vi "Lab Panel V5.27.vi"() -> ()   [LabVIEW 2013] (continued)
                    n2201 = Unbundle By Name(w3868) -> ("OFF amps"=w3864:dbl, "VOLTS"=w3863:dbl, "PF"=w3862:dbl, "OFF amps"=w3861:dbl, "VOLTS"=w3860:dbl, "PF"=w3859:dbl)
                    n2202 = Unbundle By Name(w3865) -> ("1  (A) cal"=w3858:dbl, "1 (V) cal"=w3857:dbl, "1 (PF) cal"=w3856:dbl, "2 (A) cal"=w3855:dbl, "2 (V) cal"=w3854:dbl, "2 (PF) cal"=w3853:dbl)  [unwired: 4 out]
                    n2203 = Multiply(x=w3864, y=w3858) -> (x*y=w3851:dbl)
                    n2204 = Multiply(x=w3863, y=w3857) -> (x*y=w3850:dbl)
                    n2205 = Multiply(x=w3862, y=w3856) -> (x*y=w3849:dbl)
                    n2206 = Multiply(x=w3861, y=w3855) -> (x*y=w3847:dbl)
                    n2207 = Multiply(x=w3860, y=w3854) -> (x*y=w3846:dbl)
                    n2208 = Multiply(x=w3859, y=w3853) -> (x*y=w3845:dbl)
                    n2209 = local read "SIG LAB01-1"() -> (w3852:T2)
                    n2210 = local read "SIG LAB01-2"() -> (w3848:T2)
                    n2211 = Bundle By Name(cluster=w3852, "AMPS"=w3851, "VOLTS"=w3850, "PF"=w3849) -> (w3844:T2)
                    n2212 = Bundle By Name(cluster=w3848, "AMPS"=w3847, "VOLTS"=w3846, "PF"=w3845) -> (w3843:T2)
                    n2213 = global write "Global display 1.vi" "SIG LAB01-2"(w3843) -> ()
                    n2214 = global write "Global display 1.vi" "SIG LAB01-1"(w3844) -> ()
                    n2215 = local write "SIG LAB01-2"(w3843) -> ()
                    n2216 = local write "SIG LAB01-1"(w3844) -> ()
                  }
                  frame #3 {
                    n2217 = Unbundle By Name(w3896) -> ("OFF amps"=w3892:dbl, "VOLTS"=w3891:dbl, "PF"=w3890:dbl, "OFF amps"=w3889:dbl, "VOLTS"=w3888:dbl, "PF"=w3887:dbl)
                    n2218 = case shown="True" w3895 {
                      tunnel: [w3897 w3898] -> w3893
                      tunnel: w3894 -> [_ w3898]
                      frame False {
                        n2219 = local read "CAL LAB02"() -> (w3897:T15)
                      }
                      frame True {
                      }
                    }
                    n2220 = Unbundle By Name(w3893) -> ("1  (A) cal"=w3886:dbl, "1 (V) cal"=w3885:dbl, "1 (PF) cal"=w3884:dbl, "2 (A) cal"=w3883:dbl, "2 (V) cal"=w3882:dbl, "2 (PF) cal"=w3881:dbl)  [unwired: 4 out]
                    n2221 = Multiply(x=w3892, y=w3886) -> (x*y=w3879:dbl)
                    n2222 = Multiply(x=w3891, y=w3885) -> (x*y=w3878:dbl)
                    n2223 = Multiply(x=w3890, y=w3884) -> (x*y=w3877:dbl)
                    n2224 = Multiply(x=w3889, y=w3883) -> (x*y=w3875:dbl)
                    n2225 = Multiply(x=w3888, y=w3882) -> (x*y=w3874:dbl)
                    n2226 = Multiply(x=w3887, y=w3881) -> (x*y=w3873:dbl)
                    n2227 = local read "SIG LAB02-1"() -> (w3880:T2)
                    n2228 = local read "SIG LAB02-2"() -> (w3876:T2)
                    n2229 = Bundle By Name(cluster=w3880, "AMPS"=w3879, "VOLTS"=w3878, "PF"=w3877) -> (w3872:T2)
                    n2230 = Bundle By Name(cluster=w3876, "AMPS"=w3875, "VOLTS"=w3874, "PF"=w3873) -> (w3871:T2)
                    n2231 = global write "Global display 1.vi" "SIG LAB02-1"(w3872) -> ()
                    n2232 = local write "SIG LAB02-2"(w3871) -> ()
                    n2233 = global write "Global display 1.vi" "SIG LAB02-2"(w3871) -> ()
                    n2234 = local write "SIG LAB02-1"(w3872) -> ()
                  }
                  frame #4 {
                    n2235 = Unbundle By Name(w3924) -> ("OFF amps"=w3920:dbl, "VOLTS"=w3919:dbl, "PF"=w3918:dbl, "OFF amps"=w3917:dbl, "VOLTS"=w3916:dbl, "PF"=w3915:dbl)
                    n2236 = case shown="True" w3923 {
                      tunnel: [w3925 w3926] -> w3921
                      tunnel: w3922 -> [_ w3926]
                      frame False {
                        n2237 = local read "CAL LAB03"() -> (w3925:T14)
                      }
                      frame True {
                      }
                    }
                    n2238 = Unbundle By Name(w3921) -> ("1  (A) cal"=w3914:dbl, "1 (V) cal"=w3913:dbl, "1 (PF) cal"=w3912:dbl, "2 (A) cal"=w3911:dbl, "2 (V) cal"=w3910:dbl, "2 (PF) cal"=w3909:dbl)  [unwired: 4 out]
                    n2239 = Multiply(x=w3920, y=w3914) -> (x*y=w3907:dbl)
                    n2240 = Multiply(x=w3919, y=w3913) -> (x*y=w3901:dbl)
                    n2241 = Multiply(x=w3918, y=w3912) -> (x*y=w3906:dbl)
                    n2242 = Multiply(x=w3917, y=w3911) -> (x*y=w3904:dbl)
                    n2243 = Multiply(x=w3916, y=w3910) -> (x*y=w3903:dbl)
                    n2244 = Multiply(x=w3915, y=w3909) -> (x*y=w3902:dbl)
                    n2245 = local read "SIG LAB03-1"() -> (w3908:T2)
                    n2246 = local read "SIG LAB03-2"() -> (w3905:T2)
                    n2247 = Bundle By Name(cluster=w3908, "AMPS"=w3907, "VOLTS"=w3901, "PF"=w3906) -> (w3900:T2)
                    n2248 = Bundle By Name(cluster=w3905, "AMPS"=w3904, "VOLTS"=w3903, "PF"=w3902) -> (w3899:T2)
                    n2249 = global write "Global display 1.vi" "SIG LAB03-1"(w3900) -> ()
                    n2250 = global write "Global display 1.vi" "SIG LAB03-2"(w3899) -> ()
                    n2251 = local write "SIG LAB03-2"(w3899) -> ()
                    n2252 = local write "SIG LAB03-1"(w3900) -> ()
                  }
                  frame #5 {
                    n2253 = case shown="False" w3951 {
                      tunnel: [w3953 w3954] -> w3949
                      tunnel: w3950 -> [_ w3954]
                      frame False {
                        n2254 = local read "CAL LAB04"() -> (w3953:T14)
                      }
                      frame True {
                      }
                    }
                    n2255 = Unbundle By Name(w3952) -> ("OFF amps"=w3948:dbl, "VOLTS"=w3947:dbl, "PF"=w3946:dbl, "OFF amps"=w3945:dbl, "VOLTS"=w3944:dbl, "PF"=w3943:dbl)
                    n2256 = Unbundle By Name(w3949) -> ("1  (A) cal"=w3942:dbl, "1 (V) cal"=w3941:dbl, "1 (PF) cal"=w3940:dbl, "2 (A) cal"=w3939:dbl, "2 (V) cal"=w3938:dbl, "2 (PF) cal"=w3937:dbl)  [unwired: 4 out]
                    n2257 = Multiply(x=w3948, y=w3942) -> (x*y=w3935:dbl)
                    n2258 = Multiply(x=w3947, y=w3941) -> (x*y=w3934:dbl)
                    n2259 = Multiply(x=w3946, y=w3940) -> (x*y=w3933:dbl)
                    n2260 = Multiply(x=w3945, y=w3939) -> (x*y=w3931:dbl)
                    n2261 = Multiply(x=w3944, y=w3938) -> (x*y=w3930:dbl)
                    n2262 = Multiply(x=w3943, y=w3937) -> (x*y=w3929:dbl)
                    n2263 = local read "SIG LAB04-1"() -> (w3936:T2)
                    n2264 = local read "SIG LAB04-2"() -> (w3932:T2)
                    n2265 = Bundle By Name(cluster=w3936, "AMPS"=w3935, "VOLTS"=w3934, "PF"=w3933) -> (w3928:T2)
                    n2266 = Bundle By Name(cluster=w3932, "AMPS"=w3931, "VOLTS"=w3930, "PF"=w3929) -> (w3927:T2)
                    n2267 = global write "Global display 1.vi" "SIG LAB04-2"(w3927) -> ()
                    n2268 = global write "Global display 1.vi" "SIG LAB04-1"(w3928) -> ()
                    n2269 = local write "SIG LAB04-2"(w3927) -> ()
                    n2270 = local write "SIG LAB04-1"(w3928) -> ()
                  }
                  frame #6 {
                    n2271 = Unbundle By Name(w3980) -> ("OFF amps"=w3976:dbl, "VOLTS"=w3957:dbl, "PF"=w3975:dbl, "OFF amps"=w3974:dbl, "VOLTS"=w3973:dbl, "PF"=w3972:dbl)
                    n2272 = case shown="False" w3979 {
                      tunnel: [w3981 w3982] -> w3977
                      tunnel: w3978 -> [_ w3982]
                      frame False {
                        n2273 = local read "CAL LAB05"() -> (w3981:T14)
                      }
                      frame True {
                      }
                    }
                    n2274 = Unbundle By Name(w3977) -> ("1  (A) cal"=w3971:dbl, "1 (V) cal"=w3970:dbl, "1 (PF) cal"=w3969:dbl, "2 (A) cal"=w3968:dbl, "2 (V) cal"=w3967:dbl, "2 (PF) cal"=w3966:dbl)  [unwired: 4 out]
                    n2275 = Multiply(x=w3976, y=w3971) -> (x*y=w3964:dbl)
                    n2276 = Multiply(x=w3957, y=w3970) -> (x*y=w3963:dbl)
                    n2277 = Multiply(x=w3975, y=w3969) -> (x*y=w3962:dbl)
                    n2278 = Multiply(x=w3974, y=w3968) -> (x*y=w3960:dbl)
                    n2279 = Multiply(x=w3973, y=w3967) -> (x*y=w3959:dbl)
                    n2280 = Multiply(x=w3972, y=w3966) -> (x*y=w3958:dbl)
                    n2281 = local read "SIG LAB05-1"() -> (w3965:T2)
                    n2282 = local read "SIG LAB05-2"() -> (w3961:T2)
                    n2283 = Bundle By Name(cluster=w3965, "AMPS"=w3964, "VOLTS"=w3963, "PF"=w3962) -> (w3956:T2)
                    n2284 = Bundle By Name(cluster=w3961, "AMPS"=w3960, "VOLTS"=w3959, "PF"=w3958) -> (w3955:T2)
                    n2285 = global write "Global display 1.vi" "SIG LAB05-1"(w3956) -> ()
                    n2286 = global write "Global display 1.vi" "SIG LAB05-2"(w3955) -> ()
                    n2287 = local write "SIG LAB05-2"(w3955) -> ()
                    n2288 = local write "SIG LAB05-1"(w3956) -> ()
                  }
                  frame #7 {
                    n2289 = case shown="False" w3983 {
                      tunnel: w3985 -> [w3990 _]
                      tunnel: w3984 -> [w3989 _]
                      frame False {
                        # "update ambient referance temperature"
                        n2290 = case shown="True" w3990 {
                          tunnel: [w3992 100.0] -> w3991
                          frame False {
                            n2291 = local read "TEMP REF cal"() -> (w3992:dbl)
                          }
                          frame True {
                          }
                        }
                        n2292 = disable-structure shown="Disabled" {
                          frame Disabled {
                            n2293 = local read "Temp read loop"() -> ()  [unwired: 1 out]
                          }
                          frame Enabled {
                          }
                        }
                        n2294 = Multiply(x=w3991, y=w3989) -> (x*y=w3988:dbl)
                        n2295 = Subtract(x=w3988, y=272) -> (x-y=w3986:dbl)
                        "Amb Tp" <- w3986
                        n2296 = local write "Ref deg C"(w3986) -> ()
                        "deg C (volts)" <- w3989
                      }
                      frame True {
                      }
                    }
                  }
                }
              }
            }
          }
          frame #14 {
            # "save test data to file during testing"
            n2297 = local read "on loops"() -> (w4013:dbl)
            n2298 = Get Date/Time In Seconds() -> (seconds since 1Jan1904=w3994:timestamp)
            "File Time Stamp" <- w3994
            n2299 = local read "jig cycle"() -> (w4010:dbl)
            n2300 = Format Date/Time String(time format string (%c)="%H:%M%:%S", seconds (now)=w3994) -> (date/time string=w3998:string)  [unwired: 1 in]
            n2301 = Add(x=w4013, y=4) -> (x+y=w4011:dbl)
            n2302 = Build Array(w3998) -> (w3997:string[])
            n2303 = Equal?(x=w4010, y=3) -> (x = y?=w3996:bool)
            n2304 = Equal?(x=w4010, y=w4011) -> (x = y?=w3995:bool)
            n2305 = stacked-sequence {
              tunnel: w4009 -> [w4019 _ _ _ _ _ _ _ _ _]
              tunnel: w4008 -> [_ w4095 _ _ _ _ _ _ _ _]
              tunnel: w4007 -> [_ _ w4175 _ _ _ _ _ _ _]
              tunnel: w4006 -> [_ _ _ w4255 _ _ _ _ _ _]
              tunnel: w4005 -> [_ _ _ _ w4335 _ _ _ _ _]
              tunnel: w4004 -> [_ _ _ _ _ w4415 _ _ _ _]
              tunnel: w4003 -> [_ _ _ _ _ _ w4495 _ _ _]
              tunnel: w4002 -> [_ _ _ _ _ _ _ w4575 _ _]
              tunnel: w4001 -> [_ _ _ _ _ _ _ _ w4655 _]
              tunnel: w4000 -> [_ _ _ _ _ _ _ _ _ w4735]
              tunnel: w3997 -> [w4018 w4099 w4179 w4259 w4339 w4419 w4499 w4579 w4659 w4739]
              tunnel: w3996 -> [w4017 w4098 w4178 w4258 w4338 w4418 w4498 w4578 w4658 w4738]
              tunnel: w3995 -> [w4016 w4097 w4177 w4257 w4337 w4417 w4497 w4577 w4657 w4737]
              tunnel: w3994 -> [w4015 w4096 w4176 w4256 w4336 w4416 w4496 w4576 w4656 w4736]
              frame #0 {
                n2306 = case shown="True" w4019 {
                  tunnel: w4018 -> [_ w4024]
                  tunnel: w4017 -> [_ w4023]
                  tunnel: w4016 -> [_ w4021]
                  tunnel: w4015 -> [_ w4020]
                  frame False {
                  }
                  frame True {
                    n2307 = local read "DISP LAB01-1"() -> (w4025:T4)
                    n2308 = local read "SIG LAB01-1"() -> (w4026:T2)
                    n2309 = local read "ON L01-1"() -> (w4022:cluster{"amps":dbl, "volts":dbl, "pf":dbl})
                    n2310 = Unbundle(w4026) -> ("AMPS"=w4032:dbl, "VOLTS"=w4030:dbl, "PF"=w4029:dbl, "Tmp Live"=w4028:dbl, "Tmp Neut"=w4031:dbl)
                    n2311 = Unbundle(w4025) -> ("CYCLE"=w4027:dbl)  [unwired: 2 out]
                    n2312 = stacked-sequence {
                      tunnel: w4032 -> [w4036 w4055]
                      tunnel: w4031 -> [_ w4054]
                      tunnel: w4030 -> [w4035 w4053]
                      tunnel: w4029 -> [w4034 w4052]
                      tunnel: w4028 -> [_ w4051]
                      tunnel: w4027 -> [_ w4050]
                      tunnel: w4024 -> [_ w4049]
                      tunnel: w4023 -> [w4037 _]
                      tunnel: w4022 -> [w4033 w4047]
                      tunnel: w4021 -> [_ w4048]
                      tunnel: w4020 -> [_ w4043]
                      frame #0 {
                        n2313 = case shown="True" w4037 {
                          tunnel: w4036 -> [_ w4042]
                          tunnel: w4035 -> [_ w4041]
                          tunnel: w4034 -> [_ w4040]
                          tunnel: w4033 -> [_ w4038]
                          frame False {
                          }
                          frame True {
                            n2314 = Bundle(cluster=w4038, "amps"=w4042, "volts"=w4041, "pf"=w4040) -> (w4039:cluster{"amps":dbl, "volts":dbl, "pf":dbl})
                            n2315 = local write "ON L01-1"(w4039) -> ()
                          }
                        }
                      }
                      frame #1 {
                        n2316 = Unbundle(w4047) -> ("amps"=w4046:dbl, "volts"=w4045:dbl, "pf"=w4044:dbl)
                        n2317 = case shown="True" w4048 {
                          tunnel: w4055 -> [_ w4056]
                          tunnel: w4054 -> [_ w4094]
                          tunnel: w4053 -> [_ _]
                          tunnel: w4052 -> [_ _]
                          tunnel: w4051 -> [_ w4093]
                          tunnel: w4050 -> [_ w4092]
                          tunnel: w4049 -> [_ w4060]
                          tunnel: w4046 -> [_ w4057]
                          tunnel: w4045 -> [_ w4089]
                          tunnel: w4044 -> [_ w4088]
                          tunnel: w4043 -> [_ w4058]
                          frame False {
                          }
                          frame True {
                            n2318 = local read "TDMS LAB01-1"() -> (w4091:refnum<k34>)
                            n2319 = Build Array(w4089) -> (w4085:dbl[])
                            n2320 = Build Array(w4088) -> (w4084:dbl[])
                            n2321 = Build Array(w4093) -> (w4083:dbl[])
                            n2322 = Build Array(w4094) -> (w4082:dbl[])
                            n2323 = Build Array(w4057) -> (w4087:dbl[])
                            n2324 = Build Array(w4056) -> (w4086:dbl[])
                            n2325 = Build Array(w4092) -> (w4081:dbl[])
                            n2326 = Build Array("AMPS ON", "AMPS OFF", "VOLTS", "PF", "TEMP Live", "TEMP Neut", "CYCLE") -> (w4065:string[])
                            n2327 = Bundle By Name("Y"=w4087, "t0"=w4058) -> (w4080:waveform(dbl))  [unwired: 1 in]
                            n2328 = Bundle By Name("Y"=w4086, "t0"=w4058) -> (w4079:waveform(dbl))  [unwired: 1 in]
                            n2329 = Bundle By Name("Y"=w4085, "t0"=w4058) -> (w4078:waveform(dbl))  [unwired: 1 in]
                            n2330 = Bundle By Name("Y"=w4084, "t0"=w4058) -> (w4077:waveform(dbl))  [unwired: 1 in]
                            n2331 = Bundle By Name("Y"=w4083, "t0"=w4058) -> (w4076:waveform(dbl))  [unwired: 1 in]
                            n2332 = Bundle By Name("Y"=w4082, "t0"=w4058) -> (w4075:waveform(dbl))  [unwired: 1 in]
                            n2333 = Bundle By Name("Y"=w4081, "t0"=w4058) -> (w4074:waveform(dbl))  [unwired: 1 in]
                            n2334 = Build Array(w4080, w4079, w4078, w4077, w4076, w4075, w4074) -> (w4073:waveform(dbl)[])
                            n2335 = TDMS Write(0:w4091, 5:"TEST VALUES", 7:w4065, 9:w4073) -> (4:w4064:refnum<k34>, 6:w4063:string, 15:w4062:errorcluster)  [unwired: 2 in, 1 out]
                            n2336 = TDMS Write(0:w4064, 5:w4063, 7:"TIME", 9:w4060, 11:w4062) -> (15:w4059:errorcluster)  [unwired: 1 in, 3 out]
                            n2337 = local write "data file error"(w4059) -> ()
                          }
                        }
                      }
                    }
                  }
                }
              }
              frame #1 {
                n2338 = case shown="True" w4095 {
                  tunnel: w4099 -> [_ w4104]
                  tunnel: w4098 -> [_ w4103]
                  tunnel: w4097 -> [_ w4101]
                  tunnel: w4096 -> [_ w4100]
                  frame False {
                  }
                  frame True {
                    n2339 = local read "DISP LAB01-2"() -> (w4105:T4)
                    n2340 = local read "SIG LAB01-2"() -> (w4106:T2)
                    n2341 = local read "ON L01-2"() -> (w4102:cluster{"amps":dbl, "volts":dbl, "pf":dbl})
                    n2342 = Unbundle(w4106) -> ("AMPS"=w4112:dbl, "VOLTS"=w4110:dbl, "PF"=w4109:dbl, "Tmp Live"=w4108:dbl, "Tmp Neut"=w4111:dbl)
                    n2343 = Unbundle(w4105) -> ("CYCLE"=w4107:dbl)  [unwired: 2 out]
                    n2344 = stacked-sequence {
                      tunnel: w4112 -> [w4116 w4135]
                      tunnel: w4111 -> [_ w4134]
                      tunnel: w4110 -> [w4115 w4133]
                      tunnel: w4109 -> [w4114 w4132]
                      tunnel: w4108 -> [_ w4131]
                      tunnel: w4107 -> [_ w4130]
                      tunnel: w4104 -> [_ w4129]
                      tunnel: w4103 -> [w4117 _]
                      tunnel: w4102 -> [w4113 w4127]
                      tunnel: w4101 -> [_ w4128]
                      tunnel: w4100 -> [_ w4123]
                      frame #0 {
                        n2345 = case shown="True" w4117 {
                          tunnel: w4116 -> [_ w4122]
                          tunnel: w4115 -> [_ w4121]
                          tunnel: w4114 -> [_ w4120]
                          tunnel: w4113 -> [_ w4118]
                          frame False {
                          }
                          frame True {
                            n2346 = Bundle(cluster=w4118, "amps"=w4122, "volts"=w4121, "pf"=w4120) -> (w4119:cluster{"amps":dbl, "volts":dbl, "pf":dbl})
                            n2347 = local write "ON L01-2"(w4119) -> ()
                          }
                        }
                      }
                      frame #1 {
                        n2348 = Unbundle(w4127) -> ("amps"=w4126:dbl, "volts"=w4125:dbl, "pf"=w4124:dbl)
                        n2349 = case shown="True" w4128 {
                          tunnel: w4135 -> [_ w4167]
                          tunnel: w4134 -> [_ w4174]
                          tunnel: w4133 -> [_ _]
                          tunnel: w4132 -> [_ _]
                          tunnel: w4131 -> [_ w4173]
                          tunnel: w4130 -> [_ w4172]
                          tunnel: w4129 -> [_ w4137]
                          tunnel: w4126 -> [_ w4169]
                          tunnel: w4125 -> [_ w4168]
                          tunnel: w4124 -> [_ w4166]
                          tunnel: w4123 -> [_ w4158]
                          frame False {
                          }
                          frame True {
                            n2350 = local read "TDMS LAB01-2"() -> (w4171:refnum<k34>)
                            n2351 = Build Array(w4168) -> (w4163:dbl[])
                            n2352 = Build Array(w4166) -> (w4162:dbl[])
                            n2353 = Build Array(w4173) -> (w4161:dbl[])
                            n2354 = Build Array(w4174) -> (w4160:dbl[])
                            n2355 = Build Array(w4169) -> (w4165:dbl[])
                            n2356 = Build Array(w4167) -> (w4164:dbl[])
                            n2357 = Build Array(w4172) -> (w4159:dbl[])
                            n2358 = Build Array("AMPS ON", "AMPS OFF", "VOLTS", "PF", "TEMP Live", "TEMP Neut", "CYCLE") -> (w4142:string[])
                            n2359 = Bundle By Name("Y"=w4165, "t0"=w4158) -> (w4157:waveform(dbl))  [unwired: 1 in]
                            n2360 = Bundle By Name("Y"=w4164, "t0"=w4158) -> (w4156:waveform(dbl))  [unwired: 1 in]
                            n2361 = Bundle By Name("Y"=w4163, "t0"=w4158) -> (w4155:waveform(dbl))  [unwired: 1 in]
                            n2362 = Bundle By Name("Y"=w4162, "t0"=w4158) -> (w4154:waveform(dbl))  [unwired: 1 in]
                            n2363 = Bundle By Name("Y"=w4161, "t0"=w4158) -> (w4153:waveform(dbl))  [unwired: 1 in]
                            n2364 = Bundle By Name("Y"=w4160, "t0"=w4158) -> (w4152:waveform(dbl))  [unwired: 1 in]
                            n2365 = Bundle By Name("Y"=w4159, "t0"=w4158) -> (w4151:waveform(dbl))  [unwired: 1 in]
                            n2366 = Build Array(w4157, w4156, w4155, w4154, w4153, w4152, w4151) -> (w4150:waveform(dbl)[])
                            n2367 = TDMS Write(0:w4171, 5:"TEST VALUES", 7:w4142, 9:w4150) -> (4:w4141:refnum<k34>, 6:w4140:string, 15:w4139:errorcluster)  [unwired: 2 in, 1 out]
                            n2368 = TDMS Write(0:w4141, 5:w4140, 7:"TIME", 9:w4137, 11:w4139) -> (15:w4136:errorcluster)  [unwired: 1 in, 3 out]
                            n2369 = local write "data file error"(w4136) -> ()
                          }
                        }
                      }
                    }
                  }
                }
              }
              frame #2 {
                n2370 = case shown="True" w4175 {
                  tunnel: w4179 -> [_ w4184]
                  tunnel: w4178 -> [_ w4183]
                  tunnel: w4177 -> [_ w4181]
                  tunnel: w4176 -> [_ w4180]
                  frame False {
                  }
                  frame True {
                    n2371 = local read "DISP LAB02-1"() -> (w4185:T4)
                    n2372 = local read "SIG LAB02-1"() -> (w4186:T2)
                    n2373 = local read "ON L02-1"() -> (w4182:cluster{"amps":dbl, "volts":dbl, "pf":dbl})
                    n2374 = Unbundle(w4186) -> ("AMPS"=w4192:dbl, "VOLTS"=w4190:dbl, "PF"=w4189:dbl, "Tmp Live"=w4188:dbl, "Tmp Neut"=w4191:dbl)
                    n2375 = Unbundle(w4185) -> ("CYCLE"=w4187:dbl)  [unwired: 2 out]
                    n2376 = stacked-sequence {
                      tunnel: w4192 -> [w4196 w4215]
                      tunnel: w4191 -> [_ w4214]
                      tunnel: w4190 -> [w4195 w4213]
                      tunnel: w4189 -> [w4194 w4212]
                      tunnel: w4188 -> [_ w4211]
                      tunnel: w4187 -> [_ w4210]
                      tunnel: w4184 -> [_ w4209]
                      tunnel: w4183 -> [w4197 _]
                      tunnel: w4182 -> [w4193 w4207]
                      tunnel: w4181 -> [_ w4208]
                      tunnel: w4180 -> [_ w4203]
                      frame #0 {
                        n2377 = case shown="True" w4197 {
                          tunnel: w4196 -> [_ w4202]
                          tunnel: w4195 -> [_ w4201]
                          tunnel: w4194 -> [_ w4200]
                          tunnel: w4193 -> [_ w4198]
                          frame False {
                          }
                          frame True {
                            n2378 = Bundle(cluster=w4198, "amps"=w4202, "volts"=w4201, "pf"=w4200) -> (w4199:cluster{"amps":dbl, "volts":dbl, "pf":dbl})
                            n2379 = local write "ON L02-1"(w4199) -> ()
                          }
                        }
                      }
                      frame #1 {
                        n2380 = Unbundle(w4207) -> ("amps"=w4206:dbl, "volts"=w4205:dbl, "pf"=w4204:dbl)
                        n2381 = case shown="True" w4208 {
                          tunnel: w4215 -> [_ w4247]
                          tunnel: w4214 -> [_ w4254]
                          tunnel: w4213 -> [_ _]
                          tunnel: w4212 -> [_ _]
                          tunnel: w4211 -> [_ w4253]
                          tunnel: w4210 -> [_ w4252]
                          tunnel: w4209 -> [_ w4217]
                          tunnel: w4206 -> [_ w4249]
                          tunnel: w4205 -> [_ w4248]
                          tunnel: w4204 -> [_ w4246]
                          tunnel: w4203 -> [_ w4238]
                          frame False {
                          }
                          frame True {
                            n2382 = local read "TDMS LAB02-1"() -> (w4251:refnum<k34>)
                            n2383 = Build Array(w4248) -> (w4243:dbl[])
                            n2384 = Build Array(w4246) -> (w4242:dbl[])
                            n2385 = Build Array(w4253) -> (w4241:dbl[])
                            n2386 = Build Array(w4254) -> (w4240:dbl[])
                            n2387 = Build Array(w4249) -> (w4245:dbl[])
                            n2388 = Build Array(w4247) -> (w4244:dbl[])
                            n2389 = Build Array(w4252) -> (w4239:dbl[])
                            n2390 = Build Array("AMPS ON", "AMPS OFF", "VOLTS", "PF", "TEMP Live", "TEMP Neut", "CYCLE") -> (w4222:string[])
                            n2391 = Bundle By Name("Y"=w4245, "t0"=w4238) -> (w4237:waveform(dbl))  [unwired: 1 in]
                            n2392 = Bundle By Name("Y"=w4244, "t0"=w4238) -> (w4236:waveform(dbl))  [unwired: 1 in]
                            n2393 = Bundle By Name("Y"=w4243, "t0"=w4238) -> (w4235:waveform(dbl))  [unwired: 1 in]
                            n2394 = Bundle By Name("Y"=w4242, "t0"=w4238) -> (w4234:waveform(dbl))  [unwired: 1 in]
                            n2395 = Bundle By Name("Y"=w4241, "t0"=w4238) -> (w4233:waveform(dbl))  [unwired: 1 in]
                            n2396 = Bundle By Name("Y"=w4240, "t0"=w4238) -> (w4232:waveform(dbl))  [unwired: 1 in]
                            n2397 = Bundle By Name("Y"=w4239, "t0"=w4238) -> (w4231:waveform(dbl))  [unwired: 1 in]
                            n2398 = Build Array(w4237, w4236, w4235, w4234, w4233, w4232, w4231) -> (w4230:waveform(dbl)[])
                            n2399 = TDMS Write(0:w4251, 5:"TEST VALUES", 7:w4222, 9:w4230) -> (4:w4221:refnum<k34>, 6:w4220:string, 15:w4219:errorcluster)  [unwired: 2 in, 1 out]
                            n2400 = TDMS Write(0:w4221, 5:w4220, 7:"TIME", 9:w4217, 11:w4219) -> (15:w4216:errorcluster)  [unwired: 1 in, 3 out]
                            n2401 = local write "data file error"(w4216) -> ()
                          }
                        }
                      }
                    }
                  }
                }
              }
              frame #3 {
                n2402 = case shown="True" w4255 {
                  tunnel: w4259 -> [_ w4264]
                  tunnel: w4258 -> [_ w4263]
                  tunnel: w4257 -> [_ w4261]
                  tunnel: w4256 -> [_ w4260]
                  frame False {
                  }
                  frame True {
                    n2403 = local read "DISP LAB02-2"() -> (w4265:T4)
                    n2404 = local read "SIG LAB02-2"() -> (w4266:T2)
                    n2405 = local read "ON L02-2"() -> (w4262:cluster{"amps":dbl, "volts":dbl, "pf":dbl})
                    n2406 = Unbundle(w4266) -> ("AMPS"=w4272:dbl, "VOLTS"=w4270:dbl, "PF"=w4269:dbl, "Tmp Live"=w4268:dbl, "Tmp Neut"=w4271:dbl)
                    n2407 = Unbundle(w4265) -> ("CYCLE"=w4267:dbl)  [unwired: 2 out]
                    n2408 = stacked-sequence {
                      tunnel: w4272 -> [w4276 w4295]
                      tunnel: w4271 -> [_ w4294]
                      tunnel: w4270 -> [w4275 w4293]
                      tunnel: w4269 -> [w4274 w4292]
                      tunnel: w4268 -> [_ w4291]
                      tunnel: w4267 -> [_ w4290]
                      tunnel: w4264 -> [_ w4289]
                      tunnel: w4263 -> [w4277 _]
                      tunnel: w4262 -> [w4273 w4287]
                      tunnel: w4261 -> [_ w4288]
                      tunnel: w4260 -> [_ w4283]
                      frame #0 {
                        n2409 = case shown="True" w4277 {
                          tunnel: w4276 -> [_ w4282]
                          tunnel: w4275 -> [_ w4281]
                          tunnel: w4274 -> [_ w4280]
                          tunnel: w4273 -> [_ w4278]
                          frame False {
                          }
                          frame True {
                            n2410 = Bundle(cluster=w4278, "amps"=w4282, "volts"=w4281, "pf"=w4280) -> (w4279:cluster{"amps":dbl, "volts":dbl, "pf":dbl})
                            n2411 = local write "ON L02-2"(w4279) -> ()
                          }
                        }
                      }
                      frame #1 {
                        n2412 = Unbundle(w4287) -> ("amps"=w4286:dbl, "volts"=w4285:dbl, "pf"=w4284:dbl)
                        n2413 = case shown="True" w4288 {
                          tunnel: w4295 -> [_ w4327]
                          tunnel: w4294 -> [_ w4334]
                          tunnel: w4293 -> [_ _]
                          tunnel: w4292 -> [_ _]
                          tunnel: w4291 -> [_ w4333]
                          tunnel: w4290 -> [_ w4332]
                          tunnel: w4289 -> [_ w4297]
                          tunnel: w4286 -> [_ w4329]
                          tunnel: w4285 -> [_ w4328]
                          tunnel: w4284 -> [_ w4326]
                          tunnel: w4283 -> [_ w4318]
                          frame False {
                          }
                          frame True {
                            n2414 = local read "TDMS LAB02-2"() -> (w4331:refnum<k34>)
                            n2415 = Build Array(w4328) -> (w4323:dbl[])
                            n2416 = Build Array(w4326) -> (w4322:dbl[])
                            n2417 = Build Array(w4333) -> (w4321:dbl[])
                            n2418 = Build Array(w4334) -> (w4320:dbl[])
                            n2419 = Build Array(w4329) -> (w4325:dbl[])
                            n2420 = Build Array(w4327) -> (w4324:dbl[])
                            n2421 = Build Array(w4332) -> (w4319:dbl[])
                            n2422 = Build Array("AMPS ON", "AMPS OFF", "VOLTS", "PF", "TEMP Live", "TEMP Neut", "CYCLE") -> (w4302:string[])
                            n2423 = Bundle By Name("Y"=w4325, "t0"=w4318) -> (w4317:waveform(dbl))  [unwired: 1 in]
                            n2424 = Bundle By Name("Y"=w4324, "t0"=w4318) -> (w4316:waveform(dbl))  [unwired: 1 in]
                            n2425 = Bundle By Name("Y"=w4323, "t0"=w4318) -> (w4315:waveform(dbl))  [unwired: 1 in]
                            n2426 = Bundle By Name("Y"=w4322, "t0"=w4318) -> (w4314:waveform(dbl))  [unwired: 1 in]
                            n2427 = Bundle By Name("Y"=w4321, "t0"=w4318) -> (w4313:waveform(dbl))  [unwired: 1 in]
                            n2428 = Bundle By Name("Y"=w4320, "t0"=w4318) -> (w4312:waveform(dbl))  [unwired: 1 in]
                            n2429 = Bundle By Name("Y"=w4319, "t0"=w4318) -> (w4311:waveform(dbl))  [unwired: 1 in]
                            n2430 = Build Array(w4317, w4316, w4315, w4314, w4313, w4312, w4311) -> (w4310:waveform(dbl)[])
                            n2431 = TDMS Write(0:w4331, 5:"TEST VALUES", 7:w4302, 9:w4310) -> (4:w4301:refnum<k34>, 6:w4300:string, 15:w4299:errorcluster)  [unwired: 2 in, 1 out]
                            n2432 = TDMS Write(0:w4301, 5:w4300, 7:"TIME", 9:w4297, 11:w4299) -> (15:w4296:errorcluster)  [unwired: 1 in, 3 out]
                            n2433 = local write "data file error"(w4296) -> ()
                          }
                        }
                      }
                    }
                  }
                }
              }
              frame #4 {
                n2434 = case shown="True" w4335 {
                  tunnel: w4339 -> [_ w4344]
                  tunnel: w4338 -> [_ w4343]
                  tunnel: w4337 -> [_ w4341]
                  tunnel: w4336 -> [_ w4340]
                  frame False {
                  }
                  frame True {
                    n2435 = local read "DISP LAB03-1"() -> (w4345:T4)
                    n2436 = local read "SIG LAB03-1"() -> (w4346:T2)
                    n2437 = local read "ON L03-1"() -> (w4342:cluster{"amps":dbl, "volts":dbl, "pf":dbl})
                    n2438 = Unbundle(w4346) -> ("AMPS"=w4352:dbl, "VOLTS"=w4350:dbl, "PF"=w4349:dbl, "Tmp Live"=w4348:dbl, "Tmp Neut"=w4351:dbl)
                    n2439 = Unbundle(w4345) -> ("CYCLE"=w4347:dbl)  [unwired: 2 out]
                    n2440 = stacked-sequence {
                      tunnel: w4352 -> [w4356 w4375]
                      tunnel: w4351 -> [_ w4374]
                      tunnel: w4350 -> [w4355 w4373]
                      tunnel: w4349 -> [w4354 w4372]
                      tunnel: w4348 -> [_ w4371]
                      tunnel: w4347 -> [_ w4370]
                      tunnel: w4344 -> [_ w4369]
                      tunnel: w4343 -> [w4357 _]
                      tunnel: w4342 -> [w4353 w4367]
                      tunnel: w4341 -> [_ w4368]
                      tunnel: w4340 -> [_ w4363]
                      frame #0 {
                        n2441 = case shown="True" w4357 {
                          tunnel: w4356 -> [_ w4362]
                          tunnel: w4355 -> [_ w4361]
                          tunnel: w4354 -> [_ w4360]
                          tunnel: w4353 -> [_ w4358]
                          frame False {
                          }
                          frame True {
                            n2442 = Bundle(cluster=w4358, "amps"=w4362, "volts"=w4361, "pf"=w4360) -> (w4359:cluster{"amps":dbl, "volts":dbl, "pf":dbl})
                            n2443 = local write "ON L03-1"(w4359) -> ()
                          }
                        }
                      }
                      frame #1 {
                        n2444 = Unbundle(w4367) -> ("amps"=w4366:dbl, "volts"=w4365:dbl, "pf"=w4364:dbl)
                        n2445 = case shown="True" w4368 {
                          tunnel: w4375 -> [_ w4407]
                          tunnel: w4374 -> [_ w4414]
                          tunnel: w4373 -> [_ _]
                          tunnel: w4372 -> [_ _]
                          tunnel: w4371 -> [_ w4413]
                          tunnel: w4370 -> [_ w4412]
                          tunnel: w4369 -> [_ w4377]
                          tunnel: w4366 -> [_ w4409]
                          tunnel: w4365 -> [_ w4408]
                          tunnel: w4364 -> [_ w4406]
                          tunnel: w4363 -> [_ w4398]
                          frame False {
                          }
                          frame True {
                            n2446 = local read "TDMS LAB03-1"() -> (w4411:refnum<k34>)
                            n2447 = Build Array(w4408) -> (w4403:dbl[])
                            n2448 = Build Array(w4406) -> (w4402:dbl[])
                            n2449 = Build Array(w4413) -> (w4401:dbl[])
                            n2450 = Build Array(w4414) -> (w4400:dbl[])
                            n2451 = Build Array(w4409) -> (w4405:dbl[])
                            n2452 = Build Array(w4407) -> (w4404:dbl[])
                            n2453 = Build Array(w4412) -> (w4399:dbl[])
                            n2454 = Build Array("AMPS ON", "AMPS OFF", "VOLTS", "PF", "TEMP Live", "TEMP Neut", "CYCLE") -> (w4382:string[])
                            n2455 = Bundle By Name("Y"=w4405, "t0"=w4398) -> (w4397:waveform(dbl))  [unwired: 1 in]
                            n2456 = Bundle By Name("Y"=w4404, "t0"=w4398) -> (w4396:waveform(dbl))  [unwired: 1 in]
                            n2457 = Bundle By Name("Y"=w4403, "t0"=w4398) -> (w4395:waveform(dbl))  [unwired: 1 in]
                            n2458 = Bundle By Name("Y"=w4402, "t0"=w4398) -> (w4394:waveform(dbl))  [unwired: 1 in]
                            n2459 = Bundle By Name("Y"=w4401, "t0"=w4398) -> (w4393:waveform(dbl))  [unwired: 1 in]
                            n2460 = Bundle By Name("Y"=w4400, "t0"=w4398) -> (w4392:waveform(dbl))  [unwired: 1 in]
                            n2461 = Bundle By Name("Y"=w4399, "t0"=w4398) -> (w4391:waveform(dbl))  [unwired: 1 in]
                            n2462 = Build Array(w4397, w4396, w4395, w4394, w4393, w4392, w4391) -> (w4390:waveform(dbl)[])
                            n2463 = TDMS Write(0:w4411, 5:"TEST VALUES", 7:w4382, 9:w4390) -> (4:w4381:refnum<k34>, 6:w4380:string, 15:w4379:errorcluster)  [unwired: 2 in, 1 out]
                            n2464 = TDMS Write(0:w4381, 5:w4380, 7:"TIME", 9:w4377, 11:w4379) -> (15:w4376:errorcluster)  [unwired: 1 in, 3 out]
                            n2465 = local write "data file error"(w4376) -> ()
                          }
                        }
                      }
                    }
                  }
                }
              }
              frame #5 {
                n2466 = case shown="True" w4415 {
                  tunnel: w4419 -> [_ w4424]
                  tunnel: w4418 -> [_ w4423]
                  tunnel: w4417 -> [_ w4421]
                  tunnel: w4416 -> [_ w4420]
                  frame False {
                  }
                  frame True {
                    n2467 = local read "DISP LAB03-2"() -> (w4425:T4)
                    n2468 = local read "SIG LAB03-2"() -> (w4426:T2)
                    n2469 = local read "ON L03-2"() -> (w4422:cluster{"amps":dbl, "volts":dbl, "pf":dbl})
                    n2470 = Unbundle(w4426) -> ("AMPS"=w4432:dbl, "VOLTS"=w4430:dbl, "PF"=w4429:dbl, "Tmp Live"=w4428:dbl, "Tmp Neut"=w4431:dbl)
                    n2471 = Unbundle(w4425) -> ("CYCLE"=w4427:dbl)  [unwired: 2 out]
                    n2472 = stacked-sequence {
                      tunnel: w4432 -> [w4436 w4455]
                      tunnel: w4431 -> [_ w4454]
                      tunnel: w4430 -> [w4435 w4453]
                      tunnel: w4429 -> [w4434 w4452]
                      tunnel: w4428 -> [_ w4451]
                      tunnel: w4427 -> [_ w4450]
                      tunnel: w4424 -> [_ w4449]
                      tunnel: w4423 -> [w4437 _]
                      tunnel: w4422 -> [w4433 w4447]
                      tunnel: w4421 -> [_ w4448]
                      tunnel: w4420 -> [_ w4443]
                      frame #0 {
                        n2473 = case shown="True" w4437 {
                          tunnel: w4436 -> [_ w4442]
                          tunnel: w4435 -> [_ w4441]
                          tunnel: w4434 -> [_ w4440]
                          tunnel: w4433 -> [_ w4438]
                          frame False {
                          }
                          frame True {
                            n2474 = Bundle(cluster=w4438, "amps"=w4442, "volts"=w4441, "pf"=w4440) -> (w4439:cluster{"amps":dbl, "volts":dbl, "pf":dbl})
                            n2475 = local write "ON L03-2"(w4439) -> ()
                          }
                        }
                      }
                      frame #1 {
                        n2476 = Unbundle(w4447) -> ("amps"=w4446:dbl, "volts"=w4445:dbl, "pf"=w4444:dbl)
                        n2477 = case shown="True" w4448 {
                          tunnel: w4455 -> [_ w4487]
                          tunnel: w4454 -> [_ w4494]
                          tunnel: w4453 -> [_ _]
                          tunnel: w4452 -> [_ _]
                          tunnel: w4451 -> [_ w4493]
                          tunnel: w4450 -> [_ w4492]
                          tunnel: w4449 -> [_ w4457]
                          tunnel: w4446 -> [_ w4489]
                          tunnel: w4445 -> [_ w4488]
                          tunnel: w4444 -> [_ w4486]
                          tunnel: w4443 -> [_ w4478]
                          frame False {
                          }
                          frame True {
                            n2478 = local read "TDMS LAB03-2"() -> (w4491:refnum<k34>)
                            n2479 = Build Array(w4488) -> (w4483:dbl[])
                            n2480 = Build Array(w4486) -> (w4482:dbl[])
                            n2481 = Build Array(w4493) -> (w4481:dbl[])
                            n2482 = Build Array(w4494) -> (w4480:dbl[])
                            n2483 = Build Array(w4489) -> (w4485:dbl[])
                            n2484 = Build Array(w4487) -> (w4484:dbl[])
                            n2485 = Build Array(w4492) -> (w4479:dbl[])
                            n2486 = Build Array("AMPS ON", "AMPS OFF", "VOLTS", "PF", "TEMP Live", "TEMP Neut", "CYCLE") -> (w4462:string[])
                            n2487 = Bundle By Name("Y"=w4485, "t0"=w4478) -> (w4477:waveform(dbl))  [unwired: 1 in]
                            n2488 = Bundle By Name("Y"=w4484, "t0"=w4478) -> (w4476:waveform(dbl))  [unwired: 1 in]
                            n2489 = Bundle By Name("Y"=w4483, "t0"=w4478) -> (w4475:waveform(dbl))  [unwired: 1 in]
                            n2490 = Bundle By Name("Y"=w4482, "t0"=w4478) -> (w4474:waveform(dbl))  [unwired: 1 in]
                            n2491 = Bundle By Name("Y"=w4481, "t0"=w4478) -> (w4473:waveform(dbl))  [unwired: 1 in]
                            n2492 = Bundle By Name("Y"=w4480, "t0"=w4478) -> (w4472:waveform(dbl))  [unwired: 1 in]
                            n2493 = Bundle By Name("Y"=w4479, "t0"=w4478) -> (w4471:waveform(dbl))  [unwired: 1 in]
                            n2494 = Build Array(w4477, w4476, w4475, w4474, w4473, w4472, w4471) -> (w4470:waveform(dbl)[])
                            n2495 = TDMS Write(0:w4491, 5:"TEST VALUES", 7:w4462, 9:w4470) -> (4:w4461:refnum<k34>, 6:w4460:string, 15:w4459:errorcluster)  [unwired: 2 in, 1 out]
                            n2496 = TDMS Write(0:w4461, 5:w4460, 7:"TIME", 9:w4457, 11:w4459) -> (15:w4456:errorcluster)  [unwired: 1 in, 3 out]
                            n2497 = local write "data file error"(w4456) -> ()
                          }
                        }
                      }
                    }
                  }
                }
              }
              frame #6 {
                n2498 = case shown="True" w4495 {
                  tunnel: w4499 -> [_ w4504]
                  tunnel: w4498 -> [_ w4503]
                  tunnel: w4497 -> [_ w4501]
                  tunnel: w4496 -> [_ w4500]
                  frame False {
                  }
                  frame True {
                    n2499 = local read "DISP LAB04-1"() -> (w4505:T4)
                    n2500 = local read "SIG LAB04-1"() -> (w4506:T2)
                    n2501 = local read "ON L04-1"() -> (w4502:cluster{"amps":dbl, "volts":dbl, "pf":dbl})
                    n2502 = Unbundle(w4506) -> ("AMPS"=w4512:dbl, "VOLTS"=w4510:dbl, "PF"=w4509:dbl, "Tmp Live"=w4508:dbl, "Tmp Neut"=w4511:dbl)
                    n2503 = Unbundle(w4505) -> ("CYCLE"=w4507:dbl)  [unwired: 2 out]
                    n2504 = stacked-sequence {
                      tunnel: w4512 -> [w4516 w4535]
                      tunnel: w4511 -> [_ w4534]
                      tunnel: w4510 -> [w4515 w4533]
                      tunnel: w4509 -> [w4514 w4532]
                      tunnel: w4508 -> [_ w4531]
                      tunnel: w4507 -> [_ w4530]
                      tunnel: w4504 -> [_ w4529]
                      tunnel: w4503 -> [w4517 _]
                      tunnel: w4502 -> [w4513 w4527]
                      tunnel: w4501 -> [_ w4528]
                      tunnel: w4500 -> [_ w4523]
                      frame #0 {
                        n2505 = case shown="True" w4517 {
                          tunnel: w4516 -> [_ w4522]
                          tunnel: w4515 -> [_ w4521]
                          tunnel: w4514 -> [_ w4520]
                          tunnel: w4513 -> [_ w4518]
                          frame False {
                          }
                          frame True {
                            n2506 = Bundle(cluster=w4518, "amps"=w4522, "volts"=w4521, "pf"=w4520) -> (w4519:cluster{"amps":dbl, "volts":dbl, "pf":dbl})
                            n2507 = local write "ON L04-1"(w4519) -> ()
                          }
                        }
                      }
                      frame #1 {
                        n2508 = Unbundle(w4527) -> ("amps"=w4526:dbl, "volts"=w4525:dbl, "pf"=w4524:dbl)
                        n2509 = case shown="True" w4528 {
                          tunnel: w4535 -> [_ w4567]
                          tunnel: w4534 -> [_ w4574]
                          tunnel: w4533 -> [_ _]
                          tunnel: w4532 -> [_ _]
                          tunnel: w4531 -> [_ w4573]
                          tunnel: w4530 -> [_ w4572]
                          tunnel: w4529 -> [_ w4537]
                          tunnel: w4526 -> [_ w4569]
                          tunnel: w4525 -> [_ w4568]
                          tunnel: w4524 -> [_ w4566]
                          tunnel: w4523 -> [_ w4558]
                          frame False {
                          }
                          frame True {
                            n2510 = local read "TDMS LAB04-1"() -> (w4571:refnum<k34>)
                            n2511 = Build Array(w4568) -> (w4563:dbl[])
                            n2512 = Build Array(w4566) -> (w4562:dbl[])
                            n2513 = Build Array(w4573) -> (w4561:dbl[])
                            n2514 = Build Array(w4574) -> (w4560:dbl[])
                            n2515 = Build Array(w4569) -> (w4565:dbl[])
                            n2516 = Build Array(w4567) -> (w4564:dbl[])
                            n2517 = Build Array(w4572) -> (w4559:dbl[])
                            n2518 = Build Array("AMPS ON", "AMPS OFF", "VOLTS", "PF", "TEMP Live", "TEMP Neut", "CYCLE") -> (w4542:string[])
                            n2519 = Bundle By Name("Y"=w4565, "t0"=w4558) -> (w4557:waveform(dbl))  [unwired: 1 in]
                            n2520 = Bundle By Name("Y"=w4564, "t0"=w4558) -> (w4556:waveform(dbl))  [unwired: 1 in]
                            n2521 = Bundle By Name("Y"=w4563, "t0"=w4558) -> (w4555:waveform(dbl))  [unwired: 1 in]
                            n2522 = Bundle By Name("Y"=w4562, "t0"=w4558) -> (w4554:waveform(dbl))  [unwired: 1 in]
                            n2523 = Bundle By Name("Y"=w4561, "t0"=w4558) -> (w4553:waveform(dbl))  [unwired: 1 in]
                            n2524 = Bundle By Name("Y"=w4560, "t0"=w4558) -> (w4552:waveform(dbl))  [unwired: 1 in]
                            n2525 = Bundle By Name("Y"=w4559, "t0"=w4558) -> (w4551:waveform(dbl))  [unwired: 1 in]
                            n2526 = Build Array(w4557, w4556, w4555, w4554, w4553, w4552, w4551) -> (w4550:waveform(dbl)[])
                            n2527 = TDMS Write(0:w4571, 5:"TEST VALUES", 7:w4542, 9:w4550) -> (4:w4541:refnum<k34>, 6:w4540:string, 15:w4539:errorcluster)  [unwired: 2 in, 1 out]
                            n2528 = TDMS Write(0:w4541, 5:w4540, 7:"TIME", 9:w4537, 11:w4539) -> (15:w4536:errorcluster)  [unwired: 1 in, 3 out]
                            n2529 = local write "data file error"(w4536) -> ()
                          }
                        }
                      }
                    }
                  }
                }
              }
              frame #7 {
                n2530 = case shown="True" w4575 {
                  tunnel: w4579 -> [_ w4584]
                  tunnel: w4578 -> [_ w4583]
                  tunnel: w4577 -> [_ w4581]
                  tunnel: w4576 -> [_ w4580]
                  frame False {
                  }
                  frame True {
                    n2531 = local read "DISP LAB04-2"() -> (w4585:T4)
                    n2532 = local read "SIG LAB04-2"() -> (w4586:T2)
                    n2533 = local read "ON L04-2"() -> (w4582:cluster{"amps":dbl, "volts":dbl, "pf":dbl})
                    n2534 = Unbundle(w4586) -> ("AMPS"=w4592:dbl, "VOLTS"=w4590:dbl, "PF"=w4589:dbl, "Tmp Live"=w4588:dbl, "Tmp Neut"=w4591:dbl)
                    n2535 = Unbundle(w4585) -> ("CYCLE"=w4587:dbl)  [unwired: 2 out]
                    n2536 = stacked-sequence {
                      tunnel: w4592 -> [w4596 w4615]
